vi "DriveStraightTargetCommand.vi"(7 "Navx Target":dbl, 8 "speed":dbl=0.5, 9 "Fwd Bwd":dbl, 10 "Delay ms":u32=500, 11 "distance":dbl) -> ()   [LabVIEW 2015]
uses:
  Team Code/Robot Global Data.vi
  NavX/navX Library v2/navX Library v2.lvlib
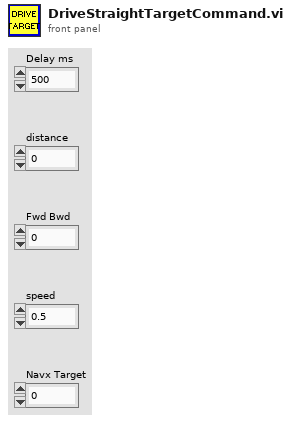
[diagram p1: front panel]
types:
  T1 = typedef "navX Library v2.lvlib/Z900_navX_DeviceTypeDef.ctl" = cluster{"Interface":cluster{"Protocol":T2, "Update Rate (4Hz-60Hz)":u8, "navX Open TypeDef":variant}, "Notify Packet":refnum<notifier>, "Loop VI Refnum":refnum<vi>, "Ready to Close Occurrence Refnum":refnum<k4>}
  T2 = typedef "navX Library v2.lvlib/Z900_navX_ProtocolTypeDef.ctl" = enum16{"SERIAL", "I2C", "SPI"}
  T3 = cluster{"Yaw":dbl, "Roll":dbl, "Pitch":dbl, "Heading":dbl, "Fused Heading":dbl}
  T4 = typedef "WPI_EncoderDevRef.ctl" = cluster{"DevStatus":errorcluster, "EncoderIndex":T5, "CounterIndex":T6, "DistancePerCount":dbl, "Decoding Type":T7}
  T5 = typedef "FPGA_EncoderIdx.ctl" = enum8{"Enc 0", "Enc 1", "Enc 2", "Enc 3", "Enc 4", "Enc 5", "Enc 6", "Enc 7", "Invalid"}
  T6 = typedef "FPGA_CounterCtrSystemIndex.ctl" = enum8{"Ctr 0", "Ctr 1", "Ctr 2", "Ctr 3", "Ctr 4", "Ctr 5", "Ctr 6", "Ctr 7", "Invalid"}
  T7 = typedef "WPI_EncoderType.ctl" = enum16{"1x", "2x", "4x"}
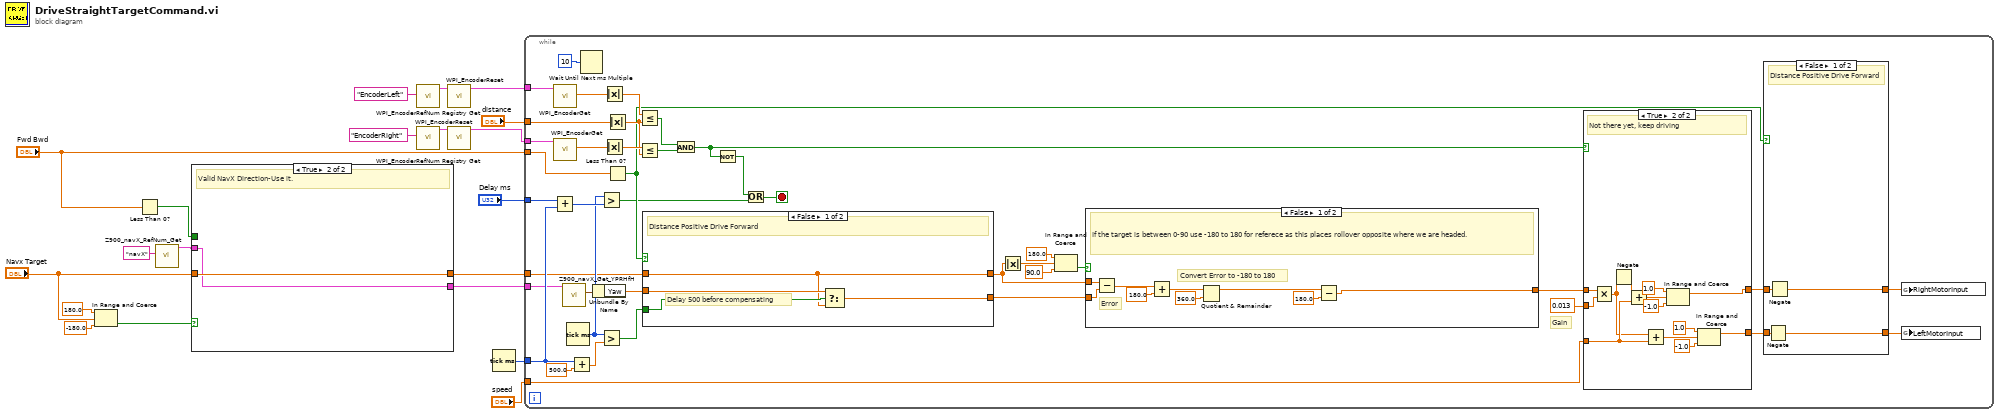
[diagram p0: block diagram]
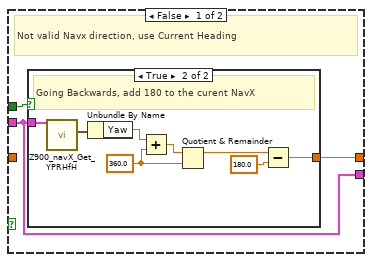
[diagram p2: hidden frame]
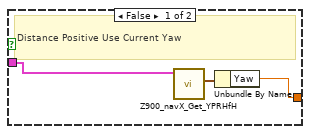
[diagram p3: hidden frame]
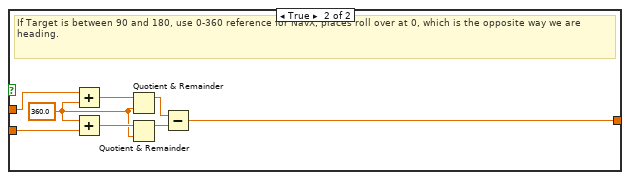
[diagram p4: hidden frame]
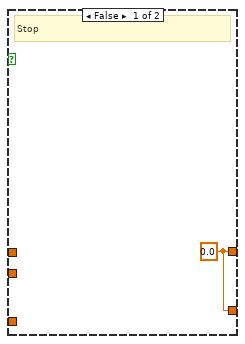
[diagram p5: hidden frame]
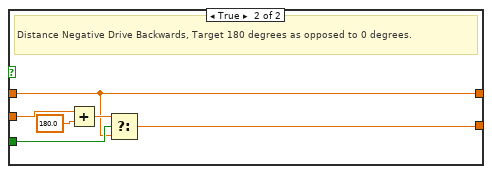
[diagram p7: hidden frame]
diagram:
  n1 = In Range and Coerce(upper limit=180.0, x="Navx Target", lower limit=-180.0) -> (In Range?=w10:bool)  [unwired: 1 out]
  n2 = Less Than 0?(x="Fwd Bwd") -> (x < 0?=w5:bool)
  n3 = call "Z900_navX_RefNum_Get.vi"("refnum name"="navX") -> ("navX Device"=w1:T1)  [unwired: 9 in, 1 out]
  n4 = case shown="True" w10 {
    tunnel: "Navx Target" -> [_ w36]
    tunnel: [w23 w36] -> w8
    tunnel: w5 -> [w22 _]
    tunnel: w1 -> [w21 w35]
    tunnel: [w21 w35] -> w3
    frame False {
      # "Not valid Navx direction, use Current Heading"
      n5 = case shown="True" w22 {
        tunnel: [w25 w30] -> w23
        tunnel: w21 -> [w24 w28]
        frame False {
          # "Distance Positive Use Current Yaw"
          n6 = call "Z900_navX_Get_YPRHfH.vi"("navX Device"=w24) -> ("YRPHfH"=w26:T3)  [unwired: 7 in, 3 out]
          n7 = Unbundle By Name(w26) -> ("Yaw"=w25:dbl)
        }
        frame True {
          w31 = 360.0 ("y")
          # "Going Backwards, add 180 to the curent NavX"
          n8 = call "Z900_navX_Get_YPRHfH.vi"("navX Device"=w28) -> ("YRPHfH"=w29:T3)  [unwired: 7 in, 3 out]
          n9 = Unbundle By Name(w29) -> ("Yaw"=w27:dbl)
          n10 = Add(x=w27, y=w31) -> (x+y=w32:dbl)
          n11 = Quotient & Remainder(x=w32, y=w31) -> (x-y*floor(x/y)=w33:dbl)  [unwired: 1 out]
          n12 = Subtract(x=w33, y=180.0) -> (x-y=w30:dbl)
        }
      }
    }
    frame True {
      # "Valid NavX Direction-Use it."
    }
  }
  n13 = call <vilib>:"WPI_EncoderRefNum Registry Get.vi"("refnum name"="EncoderLeft") -> ("EncoderDevRef"=w19:T4)  [unwired: 9 in, 1 out]
  n14 = call <vilib>:"WPI_EncoderRefNum Registry Get.vi"("refnum name"="EncoderRight") -> ("EncoderDevRef"=w18:T4)  [unwired: 9 in, 1 out]
  n15 = call <vilib>:"WPI_EncoderReset.vi"("EncoderDevRef"=w19) -> ("EncoderDevRef"=w15:T4)  [unwired: 9 in, 1 out]
  n16 = call <vilib>:"WPI_EncoderReset.vi"("EncoderDevRef"=w18) -> ("EncoderDevRef"=w14:T4)  [unwired: 9 in, 1 out]
  n17 = Tick Count (ms)() -> (millisecond timer value=w12:u32)
  n18 = while {
    tunnel: "speed" -> [w52]
    tunnel: "distance" -> [w69]
    tunnel: w15 -> [w72]
    tunnel: w14 -> [w71]
    tunnel: "Delay ms" -> [w62]
    tunnel: w12 -> [w60]
    tunnel: w8 -> [w53]
    tunnel: "Fwd Bwd" -> [w40]
    tunnel: w3 -> [w38]
    stop <- w70 stop-if-true
    # "Gain"
    n19 = call <vilib>:"WPI_EncoderGet.vi"("EncoderDevRef"=w72) -> ("Distance"=w73:dbl)  [unwired: 5 in, 5 out]
    n20 = call <vilib>:"WPI_EncoderGet.vi"("EncoderDevRef"=w71) -> ("Distance"=w74:dbl)  [unwired: 5 in, 5 out]
    n21 = Add(x=w62, y=w60) -> (x+y=w64:u32)
    n22 = call "Z900_navX_Get_YPRHfH.vi"("navX Device"=w38) -> ("YRPHfH"=w39:T3)  [unwired: 7 in, 3 out]
    n23 = Tick Count (ms)() -> (millisecond timer value=w58:u32)
    n24 = Add(x=w60, y=500.0) -> (x+y=w59:dbl)
    n25 = Wait Until Next ms Multiple(millisecond multiple=u32 10 ("milliseconds to wait")) -> ()  [unwired: 1 out]
    n26 = Unbundle By Name(w39) -> ("Yaw"=w37:dbl)
    n27 = Greater?(x=w58, y=w64) -> (0:w63:bool)
    n28 = Greater?(x=w58, y=w59) -> (0:w57:bool)
    n29 = Absolute Value(x=w73) -> (abs(x)=w75:dbl)
    n30 = Absolute Value(x=w74) -> (abs(x)=w77:dbl)
    n31 = Absolute Value(x=w69) -> (abs(x)=w76:dbl)
    n32 = Less Than 0?(x=w40) -> (x < 0?=w67:bool)
    n33 = Less Or Equal?(x=w75, y=w76) -> (x <= y?=w56:bool)
    n34 = Less Or Equal?(x=w77, y=w76) -> (x <= y?=w55:bool)
    n35 = case shown="False" w67 {
      tunnel: w37 -> [w118 w124]
      tunnel: [w117 w121] -> w41
      tunnel: [w115 w119] -> w42
      tunnel: w57 -> [w116 w120]
      tunnel: w53 -> [w115 w119]
      frame False {
        # "Delay 500 before compensating"
        # "Distance Positive Drive Forward"
        n36 = Select(t=w118, s=w116, f=w115) -> (s? t:f=w117:dbl)
      }
      frame True {
        # "Distance Negative Drive Backwards, Target 180 degrees as opposed to 0 degrees."
        n37 = Add(x=w124, y=180.0) -> (x+y=w122:dbl)
        n38 = Select(t=w122, s=w120, f=w119) -> (s? t:f=w121:dbl)
      }
    }
    n39 = And(x=w56, y=w55) -> (x .and. y?=w50:bool)
    n40 = Not(x=w50) -> (.not. x?=w54:bool)
    n41 = Or(x=w54, y=w63) -> (x .or. y?=w70:bool)
    n42 = Absolute Value(x=w42) -> (abs(x)=w45:dbl)
    n43 = In Range and Coerce(upper limit=180.0, x=w45, lower limit=90.0) -> (In Range?=w43:bool)  [unwired: 1 out]
    n44 = case shown="False" w43 {
      tunnel: [w80 w89] -> w44
      tunnel: w42 -> [w79 w94]
      tunnel: w41 -> [w78 w93]
      frame False {
        # "Convert Error to -180 to 180"
        # "Error"
        # "If the target is between 0-90 use -180 to 180 for referece as this places rollover opposite where we are headed."
        n45 = Subtract(x=w79, y=w78) -> (x-y=w81:dbl)
        n46 = Add(x=w81, y=180.0) -> (x+y=w83:dbl)
        n47 = Quotient & Remainder(x=w83, y=360.0) -> (x-y*floor(x/y)=w85:dbl)  [unwired: 1 out]
        n48 = Subtract(x=w85, y=180.0) -> (x-y=w80:dbl)
      }
      frame True {
        w90 = 360.0 ("y")
        # "If Target is between 90 and 180, use 0-360 reference for NavX, places roll over at 0, which is the opposite way we are heading."
        n49 = Add(x=w94, y=w90) -> (x+y=w92:dbl)
        n50 = Add(x=w90, y=w93) -> (x+y=w91:dbl)
        n51 = Quotient & Remainder(x=w92, y=w90) -> (x-y*floor(x/y)=w88:dbl)  [unwired: 1 out]
        n52 = Quotient & Remainder(x=w91, y=w90) -> (x-y*floor(x/y)=w87:dbl)  [unwired: 1 out]
        n53 = Subtract(x=w88, y=w87) -> (x-y=w89:dbl)
      }
    }
    n54 = case shown="True" w50 {
      tunnel: w52 -> [_ w102]
      tunnel: 0.013 ("Kp Gain") -> [_ w101]
      tunnel: [w95 w100] -> w48
      tunnel: [w95 w99] -> w49
      tunnel: w44 -> [_ w98]
      frame False {
        w95 = 0.0
        # "Stop"
      }
      frame True {
        # "Not there yet, keep driving"
        n55 = Multiply(x=w98, y=w101) -> (x*y=w97:dbl)
        n56 = Negate(x=w97) -> (-x=w96:dbl)
        n57 = Add(x=w96, y=w102) -> (x+y=w106:dbl)
        n58 = Add(x=w97, y=w102) -> (x+y=w103:dbl)
        n59 = In Range and Coerce(upper limit=1.0, x=w106, lower limit=-1.0) -> (coerced(x)=w100:dbl)  [unwired: 1 out]
        n60 = In Range and Coerce(upper limit=1.0, x=w103, lower limit=-1.0) -> (coerced(x)=w99:dbl)  [unwired: 1 out]
      }
    }
    n61 = case shown="False" w67 {
      tunnel: [w109 w114] -> w66
      tunnel: [w110 w113] -> w65
      tunnel: w49 -> [w112 w113]
      tunnel: w48 -> [w111 w114]
      frame False {
        # "Distance Positive Drive Forward"
        n62 = Negate(x=w112) -> (-x=w109:dbl)
        n63 = Negate(x=w111) -> (-x=w110:dbl)
      }
      frame True {
        # "Distance Negative, Reverse and Left becomes Right and Right Becomes Left"
      }
    }
    n64 = global write "Robot Global Data.vi" "RightMotorInput"(w65) -> ()
    n65 = global write "Robot Global Data.vi" "LeftMotorInput"(w66) -> ()
  }
